vi "Global Arm Variables.vi"() -> ()   [LabVIEW 2017]
panel:
  in  "Winch or Arm":bool
  out "illegalRangeForExtendedArm":bool
  in  "armEncoderRate":dbl
  in  "armEncoderDirection":bool
  in  "armEncoderDistance":dbl
  in  "maxAllowedLengthDuringMatch (in)":dbl
  in  "maxAllowedLengthAtStart (in)":dbl
  in  "maxAllowedFrameExtension (in)":dbl=16.0
  in  "armAngle (pot value)":dbl
  in  "Arm PID gains":T1={"proportional gain (Kc)"=13.0, "integral time (Ti, min)"=0.0001, "derivative time (Td, min)"=0.0} {"proportional gain (Kc)" min=0.0 max=15.0 step=0.01}
  in  "currentArmAngle (pot value)":dbl
  in  "potValueForArmAtZeroDegrees (pot value)":dbl=0.4
  in  "gainForJoystickControlOfPot":dbl=0.01 min=0.0 max=1.0 step=0.0001
  in  "simulatedJoystick":dbl min=-1.0 max=1.0 step=0.01
  in  "armAngle (degrees)":dbl=-30.0
  in  "frameLength (inches)":dbl=31.0
  in  "gripperLength (inches)":dbl=10.0
  in  "gripperAngle (degrees)":dbl=45.0
  in  "armJointPosition (inches)":dbl=3.0
  in  "armExtension (inches)":dbl=24.0
  in  "arm Length (inches)":dbl=30.0
  in  "potArmSetpoint (pot value)":dbl=0.495 min=0.0 max=0.6 step=0.001
  in  "simulatedArmPot":dbl=0.4 min=0.0 max=1.0 step=0.01
  # "Arm Parameters"
  # "True for Winch\nFalse for Arm"
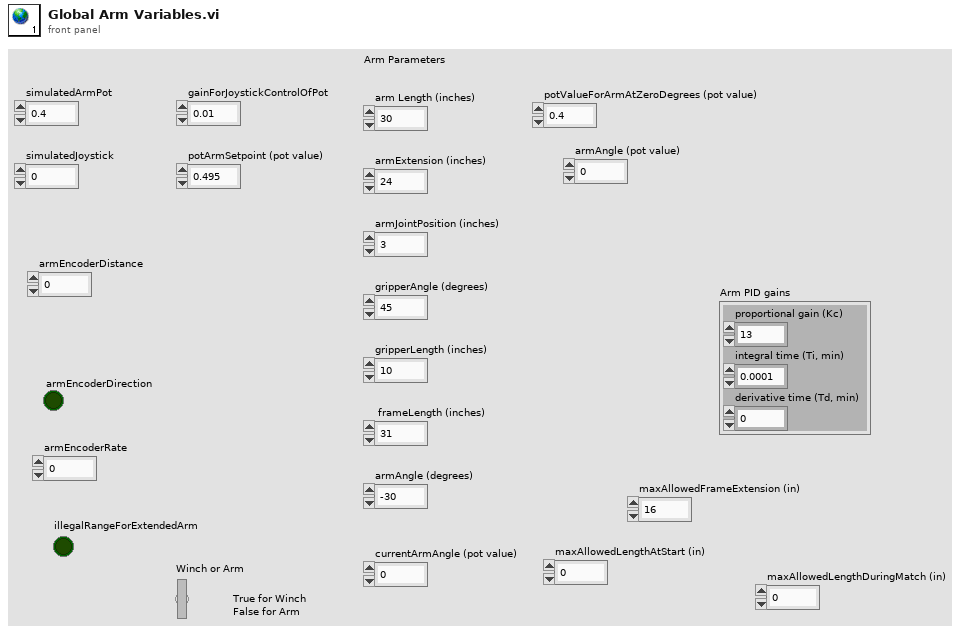
[diagram p1: front panel]
types:
  T1 = cluster{"proportional gain (Kc)":dbl, "integral time (Ti, min)":dbl, "derivative time (Td, min)":dbl}
diagram:
